vi "Auto Move Straight.vi"(6 "Target Angle":dbl, 7 "Target Distance":dbl=15.0 format="%#_13g", 8 "Error In":errorcluster, 11 "Refnum's In":T1) -> (0 "Error Out":errorcluster, 3 "Refnum's Out":T1)   [LabVIEW 2017]
uses:
  <vilib>/Rock Robotics/WPI/MotorControl/WPI_MotorControlDeviceRef.ctl
  <vilib>/Rock Robotics/WPI/MotorControl/WPI_MotorControlType.ctl
  <vilib>/Rock Robotics/SystemInterfaces/DIO/FPGA_DIOPWMChannel.ctl
  <vilib>/Rock Robotics/WPI/PWM/WPI_PWMDeadband.ctl
  <vilib>/Rock Robotics/SystemInterfaces/DIO/FPGA_DIOChannel.ctl
  <vilib>/Rock Robotics/WPI/ThirdParty/Phoenix-LabVIEW/Motor Controller/Get/CTRE_Phoenix_MotorController_GetSelectedSensorData.vi
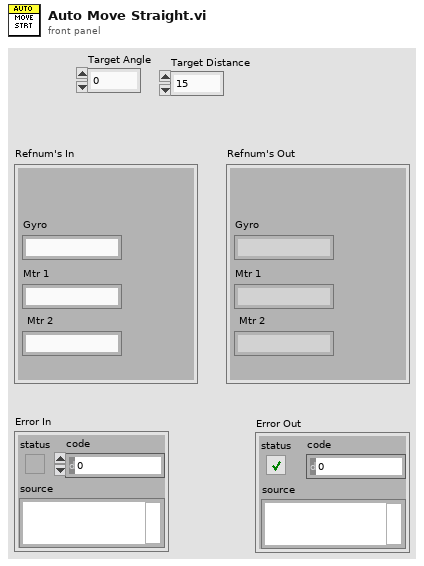
[diagram p1: front panel]
types:
  T1 = cluster{"Gyro":string, "Mtr 1":string, "Mtr 2":string}
  T2 = typedef "WPI_MotorControlDeviceRef.ctl" = cluster{"DeviceStatus":errorcluster, "Type":T3, "PWM":cluster{"PWM Channel":T4, "DeadBand":T5}, "CAN":cluster{"Device Number":u8, "SetOutput VI Ref":variant, "GetOutput VI Ref":variant, "Enable VI Ref":variant, "Disable VI Ref":variant, "Data":variant}, "Invert":bool, "DIO PWM":cluster{"PWM \"Enable\" Channel":T4, "DIOChannel":T6, "PWM Rate":dbl}}
  T3 = typedef "WPI_MotorControlType.ctl" = enum16{"PWM", "CAN", "DIO PWM"}
  T4 = typedef "FPGA_DIOPWMChannel.ctl" = enum8{"PWM 0", "PWM 1", "PWM 2", "PWM 3", "PWM 4", "PWM 5", "PWM 6", "PWM 7", "PWM 8", "PWM 9", "PWM MXP 0", "PWM MXP 1", "PWM MXP 2", "PWM MXP 3", "PWM MXP 4", "PWM MXP 5", "PWM MXP 6", "PWM MXP 7", "PWM MXP 8", "PWM MXP 9", "Invalid"}
  T5 = typedef "WPI_PWMDeadband.ctl" = cluster{"Name":string, "maxPositivePwm":i32, "minPositivePwm":i32, "centerPwm":i32, "maxNegativePwm":i32, "minNegativePwm":i32, "angularRange":u16}
  T6 = typedef "FPGA_DIOChannel.ctl" = enum8{"DIO 0", "DIO 1", "DIO 2", "DIO 3", "DIO 4", "DIO 5", "DIO 6", "DIO 7", "DIO 8", "DIO 9", "DIO MXP 0", "DIO MXP 1", "DIO MXP 2", "DIO MXP 3", "DIO MXP 4", "DIO MXP 5", "DIO MXP 6", "DIO MXP 7", "DIO MXP 8", "DIO MXP 9", "DIO MXP 10", "DIO MXP 11", "DIO MXP 12", "DIO MXP 13", "DIO MXP 14", "DIO MXP 15", "SPI Port CS1", "SPI Port CS2", "SPI Port CS3", "SPI Port MISO", "SPI Port MOSI", "Invalid"}
  T7 = typedef "WPI_GyroDevRef.ctl" = cluster{"DevStatus":errorcluster, "Analog Channel":T8, "Gain (VoltsPerDegree/Second)":dbl, "Gyro Type":enum16{"Analog", "XRS450"}, "Handle":i32, "SPI Bus":T9, "Device Found":bool, "Sample Rate":dbl, "Calibrate On Open":bool, "Offset":dbl}
  T8 = typedef "FPGA_AIChannel.ctl" = enum8{"AI 0", "AI 1", "AI 2", "AI 3", "AI MXP 0", "AI MXP 1", "AI MXP 2", "AI MXP 3", "Invalid"}
  T9 = typedef "spi_bus.ctl" = enum16{"SPI On-Board, CS0", "SPI On-Board, CS1", "SPI On-Board, CS2", "SPI On-Board, CS3", "SPI MXP", "Invalid"}
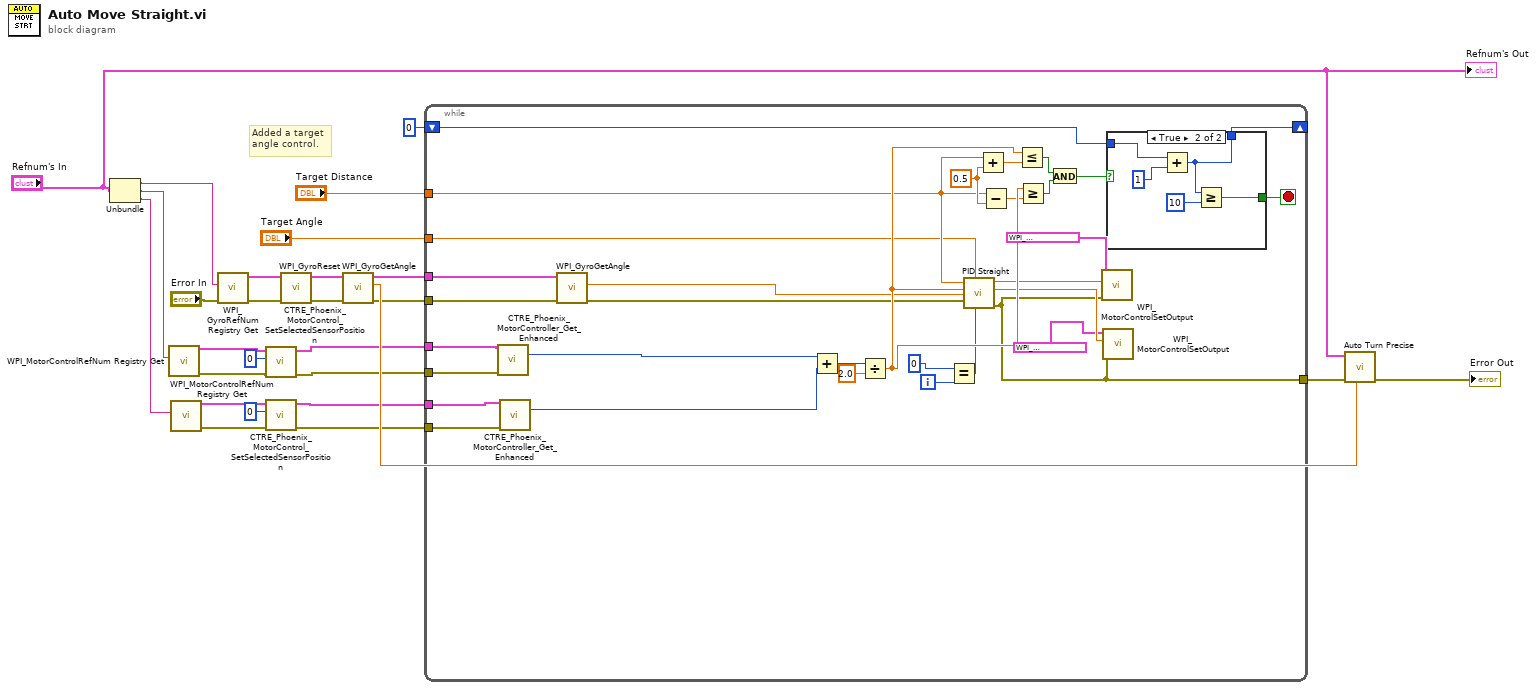
[diagram p0: block diagram]
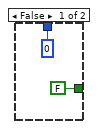
[diagram p2: hidden frame]
diagram:
  # "Added a target\nangle control."
  n1 = Unbundle("Refnum's In") -> ("Gyro"=w13:string, "Mtr 1"=w12:string, "Mtr 2"=w11:string)
  n2 = call <vilib>:"WPI_MotorControlRefNum Registry Get.vi"("refnum name"=w12) -> ("error out"=w8:errorcluster, "MotorControlDevRef"=w7:T2)  [unwired: 9 in]
  n3 = call <vilib>:"WPI_MotorControlRefNum Registry Get.vi"("refnum name"=w11) -> ("error out"=w3:errorcluster, "MotorControlDevRef"=w2:T2)  [unwired: 9 in]
  n4 = call <vilib>:"WPI_GyroRefNum Registry Get.vi"("error in (no error)"="Error In", "refnum name"=w13) -> ("error out"=w18:errorcluster, "GyroDevRef"=w17:T7)  [unwired: 8 in]
  n5 = call <vilib>:"CTRE_Phoenix_MotorControl_SetSelectedSensorPosition.vi"("error in (no error)"=w8, "New Sensor Position"=0, "PhoenixMotorControlDevRef"=w7) -> ("error out"=w9:errorcluster, "PhoenixMotorControlDevRef"=w10:T2)  [unwired: 7 in]
  n6 = call <vilib>:"CTRE_Phoenix_MotorControl_SetSelectedSensorPosition.vi"("error in (no error)"=w3, "New Sensor Position"=0, "PhoenixMotorControlDevRef"=w2) -> ("error out"=w4:errorcluster, "PhoenixMotorControlDevRef"=w5:T2)  [unwired: 7 in]
  n7 = call <vilib>:"WPI_GyroReset.vi"("error in"=w18, "GyroDevRef"=w17) -> ("error out"=w16:errorcluster, "GyroDevRef"=w15:T7)  [unwired: 8 in]
  n8 = call <vilib>:"WPI_GyroGetAngle.vi"("error in"=w16, "GyroDevRef"=w15) -> ("error out"=w20:errorcluster, "Angle"=w21:dbl, "GyroDevRef"=w19:T7)  [unwired: 5 in, 2 out]
  n9 = while {
    shift-right: [w48] -> _
    shift-left: 0 -> [w47]
    tunnel: "Target Distance" -> [w38]
    tunnel: [w30] -> w26
    tunnel: "Target Angle" -> [w37]
    tunnel: w19 -> [w40]
    tunnel: w20 -> [w39]
    tunnel: w4 -> [w35]
    tunnel: w5 -> [w36]
    tunnel: w9 -> [w32]
    tunnel: w10 -> [w33]
    i -> [w59]
    stop <- w43 stop-if-true
    w55 = 0.5 ("y")
    n10 = call-poly <vilib>:"CTRE_Phoenix_MotorController_Get_Enhanced.vi"("PhoenixMotorControlDevRef"=w33, "error in"=w32) -> ("Position (Raw Sensor Units)"=w31:i32)  [unwired: 10 in, 3 out]
    n11 = call-poly <vilib>:"CTRE_Phoenix_MotorController_Get_Enhanced.vi"("PhoenixMotorControlDevRef"=w36, "error in"=w35) -> ("Position (Raw Sensor Units)"=w34:i32)  [unwired: 10 in, 3 out]
    n12 = call <vilib>:"WPI_GyroGetAngle.vi"("error in"=w39, "GyroDevRef"=w40) -> ("error out"=w44:errorcluster, "Angle"=w46:dbl)  [unwired: 5 in, 3 out]
    n13 = Add(x=w31, y=w34) -> (x+y=w56:i32)
    n14 = Divide(x=w56, y=2.0) -> (x/y=w53:dbl)
    n15 = Equal?(x=0, y=w59) -> (x = y?=w45:bool)
    n16 = call "PID Straight.vi"("Reinitialize"=w45, "Target Angle"=w37, "Error In"=w44, "Gyro Angle"=w46, "Current Distance"=w53, "Target Distance"=w38) -> ("Error Out"=w30:errorcluster, "Right Power"=w41:dbl, "Left Power"=w42:dbl)  [unwired: 3 in]
    n17 = Add(x=w38, y=w55) -> (x+y=w54:dbl)
    n18 = Subtract(x=w38, y=w55) -> (x-y=w52:dbl)
    n19 = Less Or Equal?(x=w53, y=w54) -> (x <= y?=w51:bool)
    n20 = Greater Or Equal?(x=w53, y=w52) -> (x >= y?=w50:bool)
    n21 = And(x=w51, y=w50) -> (x .and. y?=w49:bool)
    n22 = call <vilib>:"WPI_MotorControlSetOutput.vi"("error in (no error)"=w30, "Output"=w42, "MotorControlDevRef"=T2 {"DeviceStatus"={"status"=FALSE, "code"=0, "source"=""}, "Type"=enum."PWM", "PWM"={"PWM Channel"=enum."Invalid", "DeadBand"={"Name"="", "maxPositivePwm"=0, "minPositivePwm"=0, "centerPwm"=0, "maxNegativePwm"=0, "minNegativePwm"=0, "angularRange"=0}}, "CAN"={"Device Number"=0, "SetOutput VI Ref"=variant(refnum<vi> refnum), "GetOutput VI Ref"=variant(refnum<vi> refnum), "Enable VI Ref"=variant(refnum<vi> refnum), "Disable VI Ref"=variant(refnum<vi> refnum), "Data"=variant}, "Invert"=FALSE, "DIO PWM"={"PWM \"Enable\" Channel"=enum."Invalid", "DIOChannel"=enum."Invalid", "PWM Rate"=0.0}}) -> ()  [unwired: 6 in, 3 out]
    n23 = call <vilib>:"WPI_MotorControlSetOutput.vi"("error in (no error)"=w30, "Output"=w41, "MotorControlDevRef"=T2 {"DeviceStatus"={"status"=FALSE, "code"=0, "source"=""}, "Type"=enum."PWM", "PWM"={"PWM Channel"=enum."Invalid", "DeadBand"={"Name"="", "maxPositivePwm"=0, "minPositivePwm"=0, "centerPwm"=0, "maxNegativePwm"=0, "minNegativePwm"=0, "angularRange"=0}}, "CAN"={"Device Number"=0, "SetOutput VI Ref"=variant(refnum<vi> refnum), "GetOutput VI Ref"=variant(refnum<vi> refnum), "Enable VI Ref"=variant(refnum<vi> refnum), "Disable VI Ref"=variant(refnum<vi> refnum), "Data"=variant}, "Invert"=FALSE, "DIO PWM"={"PWM \"Enable\" Channel"=enum."Invalid", "DIOChannel"=enum."Invalid", "PWM Rate"=0.0}}) -> ()  [unwired: 6 in, 3 out]
    n24 = case shown="True" w49 {
      tunnel: w47 -> [_ w65]
      tunnel: [0 w64] -> w48
      tunnel: [FALSE w62] -> w43
      frame False {
      }
      frame True {
        n25 = Add(x=w65, y=1) -> (x+y=w64:i32)
        n26 = Greater Or Equal?(x=w64, y=10) -> (x >= y?=w62:bool)
      }
    }
  }
  n27 = call "Auto Turn Precise.vi"("Target Distance"=w21, "Error In"=w26, "Refnum's In"="Refnum's In") -> ("Error Out"=→"Error Out":errorcluster)  [unwired: 7 in, 1 out]
  "Refnum's Out" <- "Refnum's In"
